vi "Stop.vi"(8 "Error In":errorcluster, 11 "object in":refnum<class "LeCroy HDO4000A.lvclass">) -> (0 "Error Out":errorcluster, 3 "object out":refnum<class "LeCroy HDO4000A.lvclass">)   [LabVIEW 2023, in "LeCroy HDO4000A.lvclass"]
uses:
  LeCroy HDO4000A.lvclass
  LeCroy HDO4000A.lvclass/LeCroy HDO4000A.ctl
  <instrlib>/LeCroy Wave Series/LeCroy Wave Series.lvlib
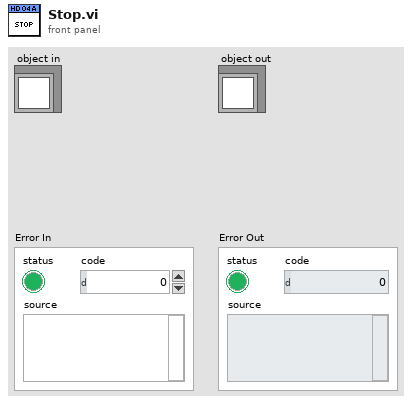
[diagram p1: front panel]
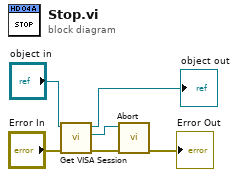
[diagram p0: block diagram]
diagram:
  n1 = call-dynamic "Get VISA Session.vi"("error in"="Error In", "Scope VISA in"="object in") -> ("error out"=w4:errorcluster, "VISA session"=w1:refnum<visa-resource-name>, "Scope VISA out"=→"object out":refnum<class "LeCroy HDO4000A.lvclass">)  [unwired: 7 in]
  n2 = call <instrlib>:"Abort.vi"("error in (no error)"=w4, "VISA resource name"=w1) -> ("error out"=→"Error Out":errorcluster)  [unwired: 8 in, 1 out]
